vi "Verwaltung Externe Stickstoff Befuellung.vi"(8 "Fehler (Eingang)":errorcluster) -> (0 "Fehler (Ausgang)":errorcluster)   [LabVIEW 2020, in "Externe Stickstoff Befuellung.lvlib"]
uses:
  Externe Stickstoff Befuellung.lvlib
  Konfig-Dateien/FGV Betriebsdaten Aktionen.ctl
  Aktionen Externe Stockstoff Befuellung.ctl
  Konfig-Dateien/Aktionen Konfig.ctl
  Konfig-Dateien/Konfig-Dateien.lvlib
  Seiten/Log Konfig/Auswahlfeld aktiviert-deaktiviert.ctl
  Seiten/Log Konfig/LogKonfig.lvlib
  Verwaltung/Verwaltung - cRIO.lvlib
  Verwaltung/FGV OUT Aktionen.ctl
panel:
  # "Verwaltung Stickstoff Befüllung"
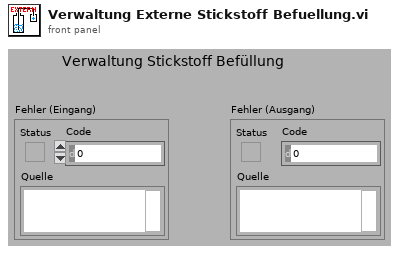
[diagram p1: front panel]
types:
  T1 = typedef "Konfig-Dateien.lvlib/FGV Betriebsdaten Aktionen.ctl" = enum16{"lesen", "Anlagengrenzw.", "PID Param.", "Sonstige", "Sensor Para."}
  T2 = typedef "Erweiterte Konfig.lvlib/Sonstige Parameter.ctl" = cluster{"Lüfter langsam":sgl, "Lüfter schnell":sgl, "FT-IR Kühlung Soll":sgl, "FT-IR Kühlung Max":sgl, "Überwachung":T3, "Befüllung aktiv":T4, "Stickstoff Befüllzeit":sgl, "Befüllintervall":sgl, "Kalibrierwert FT-IR":sgl, "Offset Ausgang":sgl, "Offset FT-IR":sgl, "Offset Druck FT-IR":sgl, "Dichtheitstest Zeit":sgl, "Dichtheitstest Abfall":sgl, "Dichtheitstest Umfang":T5, "Offset Umgebung":sgl, "Max Taupunkt":sgl, "Pumpendrehzahl":sgl, "ext. Befüllung":T4, "Ext. Stickstoff Befüllzeit":sgl}
  T3 = typedef "Auswahlfeld.ctl" = u16
  T4 = typedef "LogKonfig.lvlib/Auswahlfeld aktiviert-deaktiviert.ctl" = u16
  T5 = typedef "Erweiterte Konfig.lvlib/Dichtheitstest Umfang.ctl" = u16
  T6 = typedef "Externe Stickstoff Befuellung.lvlib/Aktionen Externe Stockstoff Befuellung.ctl" = enum16{"lesen", "Befüllen vorbereiten", "Befüllen", "Befüllen beenden", "Warten", "deaktiviert", "initialisieren"}
  T7 = typedef "Verwaltung - cRIO.lvlib/FGV OUT Aktionen.ctl" = enum16{"lesen", "ANA OUT", "DO 0-31", "DO 32-47"}
  T8 = typedef "Konfig-Dateien.lvlib/Aktionen Konfig.ctl" = enum16{"lesen", "laden", "speichern  System.ini", "speichern Anlagengrenzw.", "speichern PID + Sonstige", "speichern BSZ BMP", "speichern BSZ FT-IR", "speichern Stickstoff Bef.", "speichern Ext. Stickstoff Bef.", "speichern CAN_Konfig"}
  T9 = typedef "Verwaltung - cRIO.lvlib/Digital Ausgaenge 32-63.ctl" = cluster{"O32: Messgaspumpe EIN":bool, "O33: (Umgebungsluftpumpe)":bool, "O34: (Kondensatpumpe GK)":bool, "O35: Klima/Lüfter EIN":bool, "O36: Versorgung Heizungen":bool, "O37: Versorgung Heizungen":bool, "O38: (Gaskühler EIN (Freigabe))":bool, "O39: Störung FAS LP":bool, "O40: (Heizung Filterblock)":bool, "O41: Heizung HL zu FT-IR":bool, "O42: Heizung HL Extern SP1":bool, "O43: Heizung HL Extern SP2":bool, "O44: Heizung Reserve":bool, "O45: Heizung Reserve":bool, "O46: Statusbeleuchtung grün":bool, "O47: Statusbeleuchtung rot":bool}
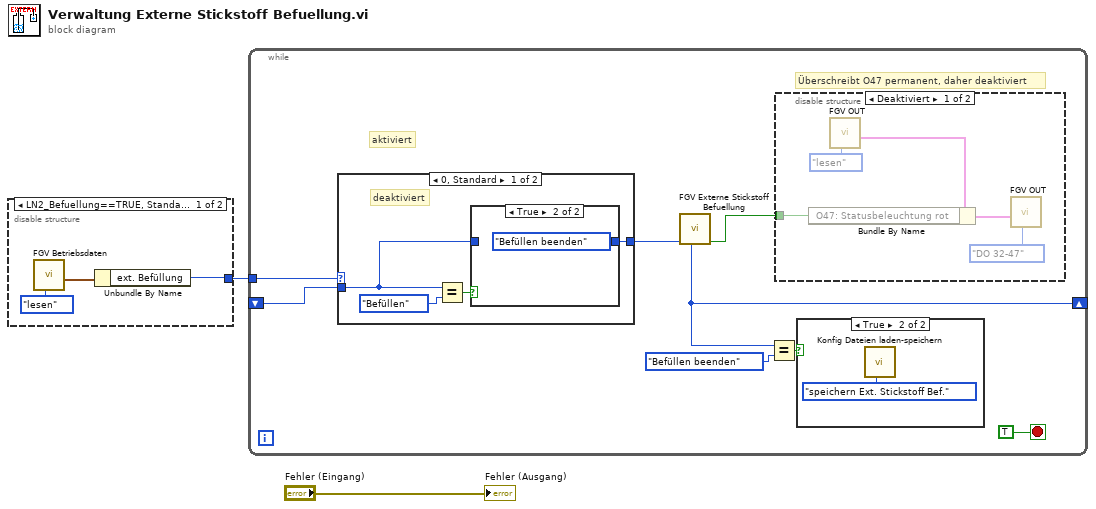
[diagram p0: block diagram]
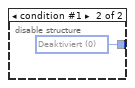
[diagram p2: hidden frame]
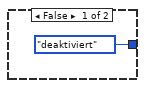
[diagram p4: hidden frame]
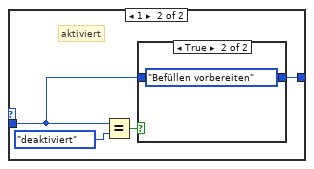
[diagram p5: hidden frame]
diagram:
  n1 = disable-structure shown="LN2_Befuellung==TRUE, Standard" {
    disable-tunnel: [w3 w6] -> w1
    frame condition #0 (active) {
      n2 = call "FGV Betriebsdaten.vi"("Aktionen"=FGV_Betriebsdaten_Aktionen."lesen") -> ("Sonstige"=w4:T2)  [unwired: 7 in, 3 out]
      n3 = Unbundle By Name(w4) -> ("ext. Befüllung"=w3:T4)
    }
    frame condition #1 {
      w6 = T4 0 items=["Deaktiviert", "Aktiviert"] ("ext. Befüllung")
    }
  }
  n4 = while {
    shift-right: [w10] -> _
    shift-left: _ -> [w13]
    tunnel: w1 -> [w8]
    stop <- TRUE stop-if-true
    # "Überschreibt O47 permanent, daher deaktiviert"
    # "aktiviert"
    n5 = case shown="0, Standard" w8 {
      tunnel: w13 -> [w21 w27]
      tunnel: [w20 w26] -> w12
      frame 0, Default {
        # "deaktiviert"
        n6 = Equal?(x=w21, y=Aktionen_Externe_Stockstoff_Befuellung."Befüllen" ("x")) -> (x = y?=w22:bool)
        n7 = case shown="True" w22 {
          tunnel: w21 -> [_ _]
          tunnel: [Aktionen_Externe_Stockstoff_Befuellung."deaktiviert" ("Aktion") Aktionen_Externe_Stockstoff_Befuellung."Befüllen beenden" ("Aktion")] -> w20
          frame False {
          }
          frame True {
          }
        }
      }
      frame 1 {
        # "aktiviert"
        n8 = Equal?(x=w27, y=Aktionen_Externe_Stockstoff_Befuellung."deaktiviert" ("x")) -> (x = y?=w28:bool)
        n9 = case shown="True" w28 {
          tunnel: w27 -> [w30 _]
          tunnel: [w30 Aktionen_Externe_Stockstoff_Befuellung."Befüllen vorbereiten" ("Aktion")] -> w26
          frame False {
          }
          frame True {
          }
        }
      }
    }
    n10 = call "FGV Externe Stickstoff Befuellung.vi"("Aktion"=w12) -> ("Ausgang"=w7:bool, "Aktion"=w10:T6)  [unwired: 4 in, 5 out]
    n11 = Equal?(x=w10, y=Aktionen_Externe_Stockstoff_Befuellung."Befüllen beenden" ("x")) -> (x = y?=w9:bool)
    n12 = disable-structure shown="Deaktiviert" {
      disable-tunnel: w7 -> [w19 _]
      frame Disabled {
        n13 = call "FGV OUT.vi"("Aktion"=FGV_OUT_Aktionen."lesen") -> ("DO 32-63"=w17:T9)  [unwired: 7 in, 3 out]
        n14 = Bundle By Name(cluster=w17, "O47: Statusbeleuchtung rot"=w19) -> (w16:T9)
        n15 = call "FGV OUT.vi"("Aktion"=FGV_OUT_Aktionen."DO 32-47", "DO 32-63"=w16) -> ()  [unwired: 6 in, 4 out]
      }
      frame Enabled {
      }
    }
    n16 = case shown="True" w9 {
      frame False {
      }
      frame True {
        n17 = call "Konfig Dateien laden-speichern.vi"("Aktion"=Aktionen_Konfig."speichern Ext. Stickstoff Bef.") -> ()  [unwired: 10 in, 1 out]
      }
    }
  }
  "Fehler (Ausgang)" <- "Fehler (Eingang)"
